vi "Configure Function.vi"(7 "Function":u16(ring) items=["DCI", "DCV"], 8 "error in (no error)":errorcluster, 11 "Agilent 344xxA in":refnum<class "Agilent 344xxA.lvclass">) -> (0 "error out":errorcluster, 3 "Agilent 344xxA out":refnum<class "Agilent 344xxA.lvclass">)   [LabVIEW 2020, in "Agilent 344xxA.lvclass"]
uses:
  Agilent 344xxA.lvclass
  C:/Sandbox/Git_Sandbox/WiSpry Test Framework source code (LV20)/WiSpry Test Framework/Instruments/Instrument.lvclass
  Instrument.lvclass/Instrument.ctl
  Instrument.lvclass
  <instrlib>/Agilent 34401/Agilent 34401.lvlib
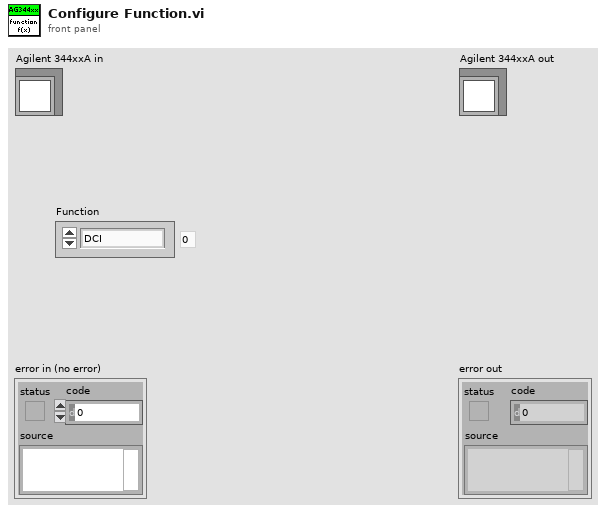
[diagram p1: front panel]
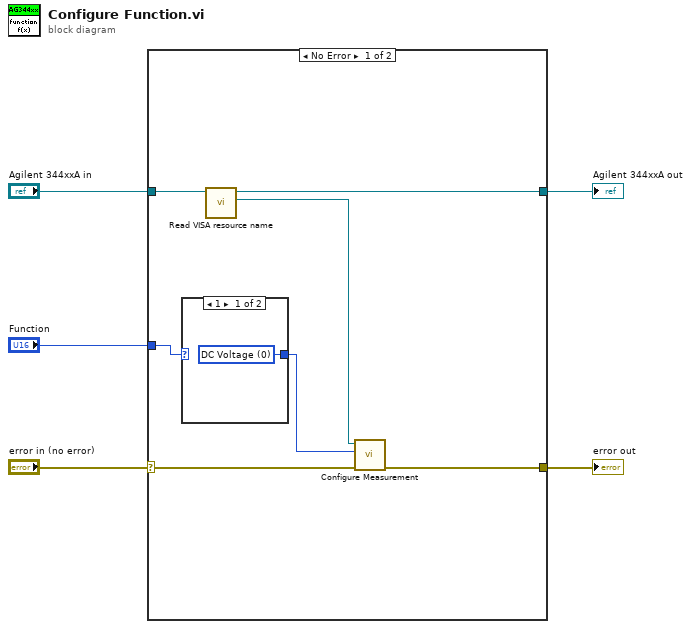
[diagram p0: block diagram]
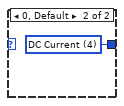
[diagram p2: hidden frame]
diagram:
  n1 = case shown="No Error" "error in (no error)" {
    selector: "error in (no error)" -> [w10 w16]
    tunnel: "Agilent 344xxA in" -> [w12 w15]
    tunnel: [w11 w15] -> w4
    tunnel: [w9 w16] -> w2
    tunnel: "Function" -> [w7 _]
    frame No Error {
      n2 = case shown="1" w7 {
        tunnel: [w13 w14] -> w6
        frame 1 {
          w13 = u16 0 items=["DC Voltage", "AC Voltage", "2 - Wire Resistance", "4 - Wire Resistance", "DC Current", "AC Current", "Frequency", "Period", "Continuity", "Diode Checking", "VDC:VDC Ratio", "Temperature", "Capacitance"] ("Function (0: DC Voltage)")
        }
        frame 0, Default {
          w14 = u16 4 items=["DC Voltage", "AC Voltage", "2 - Wire Resistance", "4 - Wire Resistance", "DC Current", "AC Current", "Frequency", "Period", "Continuity", "Diode Checking", "VDC:VDC Ratio", "Temperature", "Capacitance"] ("Function (0: DC Voltage)")
        }
      }
      n3 = call "Read VISA resource name.vi"("Instrument in"=w12) -> ("VISA resource name"=w8:refnum<visa-resource-name>, "Instrument out"=w11:refnum<class "Agilent 344xxA.lvclass">)  [unwired: 9 in]
      n4 = call <instrlib>:"Configure Measurement.vi"("error in (no error)"=w10, "Function (0: DC Voltage)"=w6, "VISA resource name"=w8) -> ("error out"=w9:errorcluster)  [unwired: 7 in, 1 out]
    }
    frame Error {
    }
  }
  "error out" <- w2
  "Agilent 344xxA out" <- w4
